vi "Integrals (SubVI).vi"(11 "Array out":dbl[](array[numeric])) -> (2 "Velocity X":dbl[](array[numeric]), 3 "Distance X":dbl[](array[numeric]))   [LabVIEW 2011]
uses:
  <vilib>/Analysis/NI_AALPro.lvlib
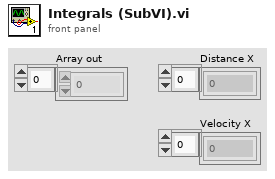
[diagram p1: front panel]
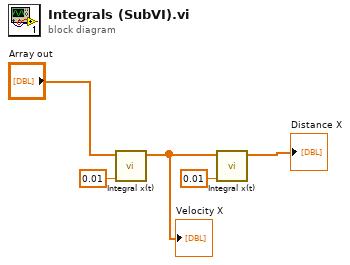
[diagram p0: block diagram]
diagram:
  n1 = call <vilib>:"Integral x(t).vi"("dt"=0.01, "X"="Array out") -> ("Integral X"=w4:dbl[])  [unwired: 8 in, 1 out]
  "Velocity X" <- w4
  n2 = call <vilib>:"Integral x(t).vi"("dt"=0.01, "X"=w4) -> ("Integral X"=→"Distance X":dbl[])  [unwired: 8 in, 1 out]
